vi "Calculate correction time.vi"(8 "error in (no error)":errorcluster) -> (3 "Correction time":dbl)   [LabVIEW 2020]
uses:
  Global Variables/General Globals.vi
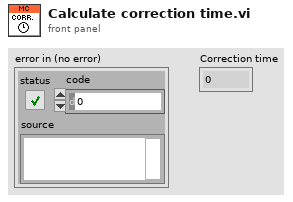
[diagram p1: front panel]
types:
  T1 = typedef "Ref DAQ Param.ctl" = cluster{"Full Frame Size":u16, "Ref Field of View":sgl, "Ref Zoom":i8, "Ref_dwellTime":sgl, "Ref X-pixels-per-line(Npxr)":i16, "Ref Y-lines-per-image(Npyr)":i16, "Ref Z-lines-per-image":i16, "Ignore Z lines":i16, "Ref Scan Cycles":i32, "Ref threshold XY":u16, "Ref threshold Z":u16, "Ref average XY":u16, "Ref Average  Z":u16, "Proportional_scale":fxp<+,16,2>, "Integral_scale":fxp<+/-,16,12>, "Proportional_scale Z":fxp<+,16,2>, "Integral_scale Z":fxp<+/-,16,12>, "Diff_threshold":fxp<+,16,2>, "Diff_threshold _z":fxp<+,16,2>, "Sliding Average":bool, "Ref count reset enabled":bool, "Auto-centering":bool}
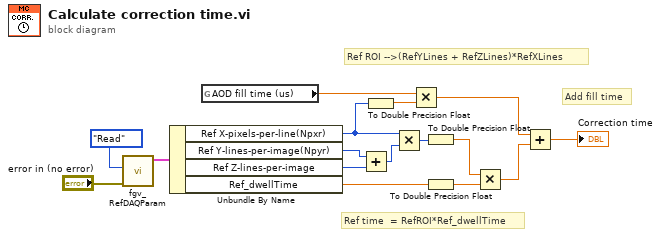
[diagram p0: block diagram]
diagram:
  # "Add fill time"
  # "Ref time  = RefROI*Ref_dwellTime"
  # "Ref ROI -->(RefYLines + RefZLines)*RefXLines"
  n1 = call "fgv_RefDAQParam.vi"("error in (no error)"="error in (no error)", "Function"=enum16{"Initialize", "Write", "Read"}."Read" ("Status")) -> ("RefDAQParam"=w3:T1)  [unwired: 8 in, 1 out]
  n2 = Unbundle By Name(w3) -> ("Ref X-pixels-per-line(Npxr)"=w12:i16, "Ref Y-lines-per-image(Npyr)"=w5:i16, "Ref Z-lines-per-image"=w4:i16, "Ref_dwellTime"=w9:sgl)
  n3 = global read "General Globals.vi" "AOD fill time (us)"() -> (w11:dbl)
  n4 = Add(x=w5, y=w4) -> (x+y=w6:i16)
  n5 = To Double Precision Float(number=w12) -> (double precision float=w13:dbl)
  n6 = Multiply(x=w12, y=w6) -> (x*y=w7:i16)
  n7 = Multiply(x=w11, y=w13) -> (x*y=w14:dbl)
  n8 = To Double Precision Float(number=w7) -> (double precision float=w8:dbl)
  n9 = To Double Precision Float(number=w9) -> (double precision float=w10:dbl)
  n10 = Multiply(x=w8, y=w10) -> (x*y=w15:dbl)
  n11 = Add(x=w14, y=w15) -> (x+y=→"Correction time":dbl)
